vi "AH2500.SHOW STATUS.vi"(8 "error in (no error)":errorcluster, 11 "VISA resource name":refnum<visa-resource-name>) -> (0 "error out":errorcluster, 2 "read buffer":string, 3 "VISA resource name out":refnum<visa-resource-name>)   [LabVIEW 2019, in "Inst.AH2500.lvclass"]
uses:
  Inst.AH2500.lvclass
panel:
  # "SHOW STATUS"
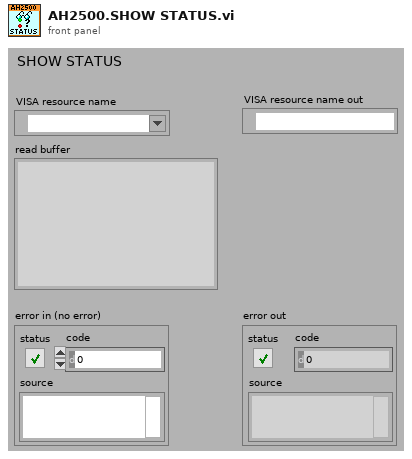
[diagram p1: front panel]
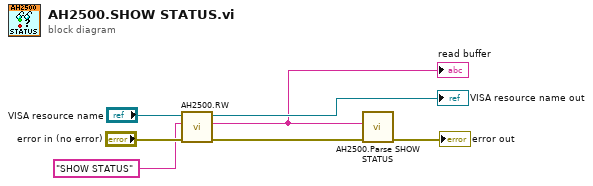
[diagram p0: block diagram]
diagram:
  n1 = call "AH2500.RW.vi"("error in (no error)"="error in (no error)", "write buffer"="SHOW STATUS", "VISA Refnum in"="VISA resource name") -> ("error out"=w2:errorcluster, "read buffer"=w1:string, "VISA Refnum out"=→"VISA resource name out":refnum<visa-resource-name>)  [unwired: 6 in]
  "read buffer" <- w1
  n2 = call "AH2500.Parse SHOW STATUS.vi"("error in"=w2, "read buffer"=w1) -> ("error out"=→"error out":errorcluster)  [unwired: 9 in]
